vi "HackRF_Driver(SubVI).vi"(8 "SampleFrequencyMHz":dbl=2.0 format="%#_13g", 9 "CarrierFrequencyMHz":dbl=104.3, 10 "Device index":i32, 11 ".NET Refnum in":refnum<k24>) -> (0 "error out":errorcluster, 2 "StartRX":refnum<k24>, 3 ".NET Refnum out":refnum<k24>)   [LabVIEW 2013]
panel:
  out "HackrfVersion":string
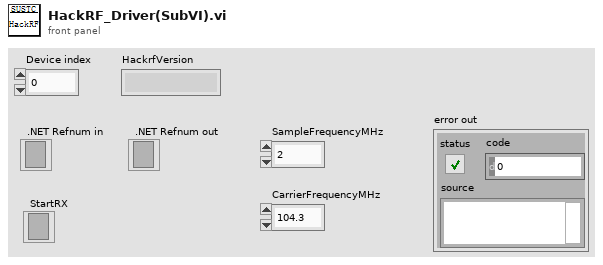
[diagram p1: front panel]
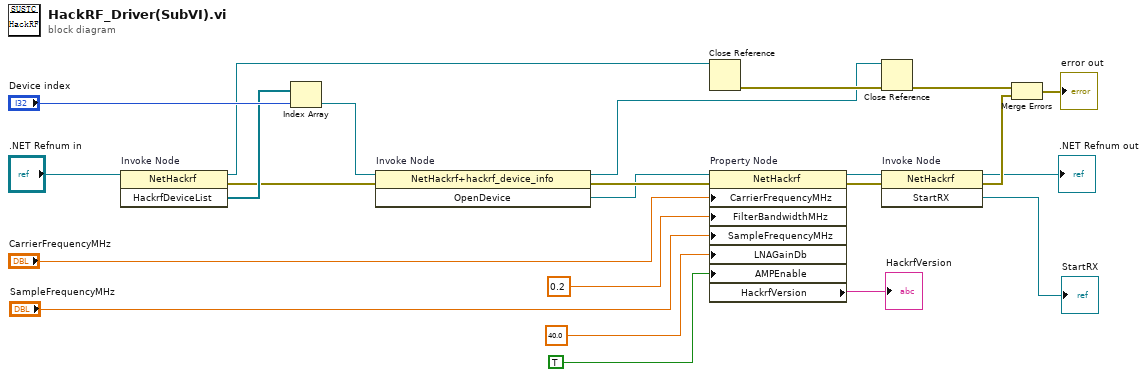
[diagram p0: block diagram]
diagram:
  n1 = invoke on="Invoke Node" class="NetHackrf" method="HackrfDeviceList"(reference=".NET Refnum in") -> (reference out=w13:refnum<k24>, error out=w4:errorcluster, "HackrfDeviceList"=w5:refnum<k24>[])  [unwired: 2 in]
  n2 = Index Array(array=w5, index="Device index") -> (element=w6:refnum<k24>)
  n3 = invoke on="Invoke Node" class="NetHackrf+hackrf_device_info" method="OpenDevice"(reference=w6, error in=w4) -> (reference out=w12:refnum<k24>, error out=w18:errorcluster, "OpenDevice"=w17:refnum<k24>)  [unwired: 1 in]
  n4 = Close Reference(reference=w13) -> (error out=w16:errorcluster)  [unwired: 1 in]
  n5 = property on="Property Node" class="NetHackrf"(reference=w17, error in=w18, "CarrierFrequencyMHz"="CarrierFrequencyMHz", "FilterBandwidthMHz"=0.2, "SampleFrequencyMHz"="SampleFrequencyMHz", "LNAGainDb"=40.0, "AMPEnable"=TRUE) -> (reference out=w7:refnum<k24>, error out=w8:errorcluster, "HackrfVersion"=→"HackrfVersion":string)
  n6 = Close Reference(reference=w12, error in (no error)=w16) -> (error out=w21:errorcluster)
  n7 = invoke on="Invoke Node" class="NetHackrf" method="StartRX"(reference=w7, error in=w8) -> (reference out=→".NET Refnum out":refnum<k24>, error out=w22:errorcluster, "StartRX"=→"StartRX":refnum<k24>)  [unwired: 1 in]
  n8 = Merge Errors(w21, w22) -> (→"error out":errorcluster)
